vi "AddManySingle.vi"(7 "Priority":refnum<class "Action.lvclass">[](array[class]), 10 "Standard":refnum<class "Action.lvclass">, 11 "ActionStack in":refnum<class "Action.lvclass">[](array[class])) -> (3 "ActionStack out":refnum<class "Action.lvclass">[](array[class]))   [LabVIEW 2024, in "ActionStack.lvlib" / "Action.lvclass"]
uses:
  Action.lvclass
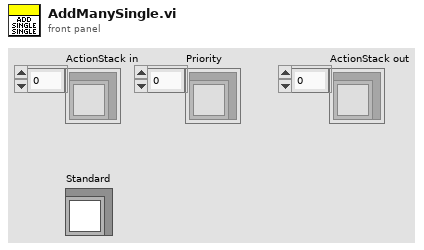
[diagram p1: front panel]
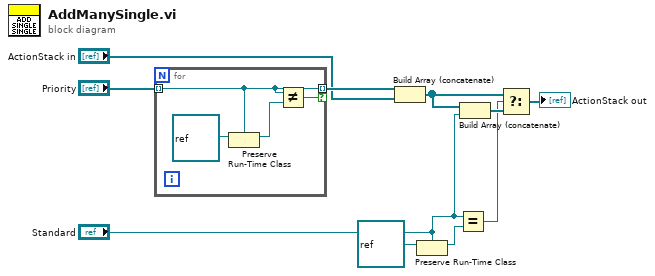
[diagram p0: block diagram]
diagram:
  n1 = for {
    tunnel: "Priority" -> [w12] mode=indexing
    tunnel: [w12] -> w3 mode=indexing if=w11
    n2 = Preserve Run-Time Class(object in=refnum<class> refnum, 2:w12) -> (object out=w13:refnum<class "Action.lvclass">)  [unwired: 1 in, 1 out]
    n3 = Not Equal?(x=w12, y=w13) -> (x != y?=w11:bool)
  }
  n4 = Build Array (concatenate)(w3, "ActionStack in") -> (w1:refnum<class "Action.lvclass">[])
  n5 = Preserve Run-Time Class(object in=refnum<class> refnum, 2:"Standard") -> (object out=w9:refnum<class "Action.lvclass">)  [unwired: 1 in, 1 out]
  n6 = Equal?(x="Standard", y=w9) -> (x = y?=w5:bool)
  n7 = Build Array (concatenate)(w1, "Standard") -> (w6:refnum<class "Action.lvclass">[])
  n8 = Select(t=w1, s=w5, f=w6) -> (s? t:f=→"ActionStack out":refnum<class "Action.lvclass">[])
